vi "Get Access Type.vi"(8 "error in":errorcluster, 11 "Object Entry in":refnum<class "Object Entry.lvclass">) -> (0 "error out":errorcluster, 2 "Access Type":T1=enum."rwr", 3 "Object Entry out":refnum<class "Object Entry.lvclass">)   [LabVIEW 2020, in "CANopen.lvlib" / "Object Entry.lvclass"]
uses:
  Object Entry.lvclass
  Object Entry.lvclass/Object Entry.ctl
  Sub Objects Dictionary/Sub Objects Dictionary.lvclass
  Sub Object/Sub Object.lvclass
  Typedefs/Access Type.ctl
  CANopen.lvlib
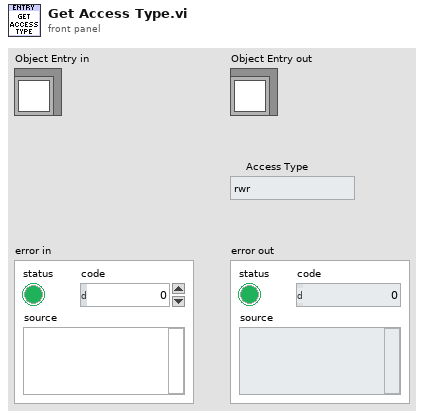
[diagram p1: front panel]
types:
  T1 = typedef "CANopen.lvlib/Access Type.ctl" = enum16{"unknown", "ro", "wo", "rw", "rwr", "rww", "const"}
  T2 = typedef "CANopen.lvlib/Object Type.ctl" = u8
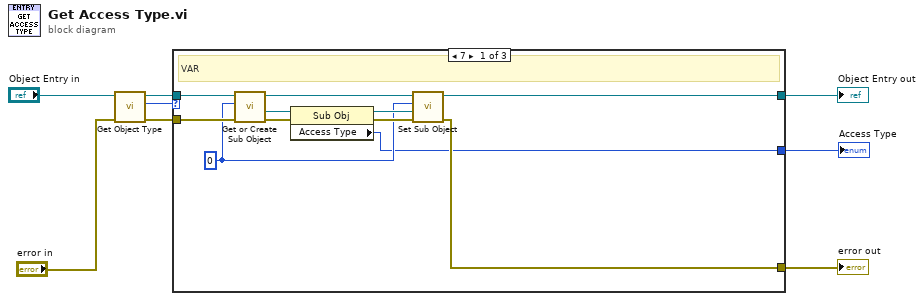
[diagram p0: block diagram]
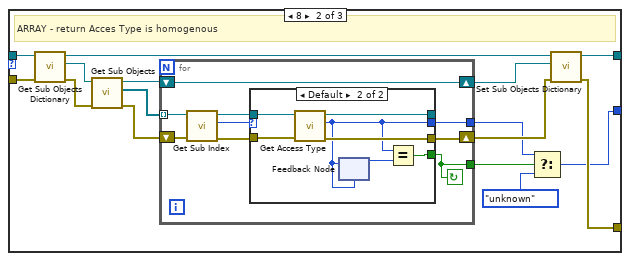
[diagram p2: hidden frame]
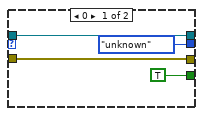
[diagram p3: hidden frame]
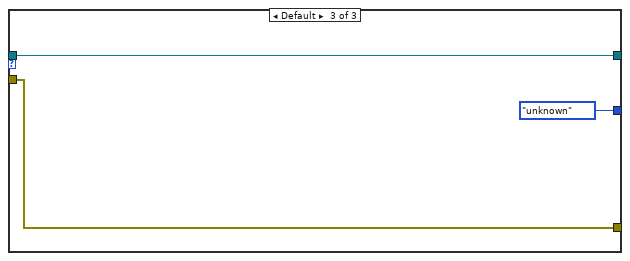
[diagram p4: hidden frame]
diagram:
  n1 = call "Get Object Type.vi"("error in"="error in", "Object Entry in"="Object Entry in") -> ("error out"=w6:errorcluster, "Object Type"=w8:T2, "Object Entry out"=w7:refnum<class "Object Entry.lvclass">)  [unwired: 7 in]
  n2 = case shown="7" w8 {
    tunnel: w7 -> [w19 w33 w57]
    tunnel: w6 -> [w16 w35 w58]
    tunnel: [w12 w24 w58] -> w1
    tunnel: [w11 w27 w57] -> w3
    tunnel: [w9 w20 Access_Type."unknown" ("f")] -> w2
    frame 7 {
      w10 = u8 0 ("Sub Index")
      # "VAR"
      n3 = call "Get or Create Sub Object.vi"("error in"=w16, "Sub Index"=w10, "Obj Entry in"=w19) -> ("error out"=w18:errorcluster, "Sub Object"=w17:refnum<class "Sub Object.lvclass">, "Obj Entry out"=w15:refnum<class "Object Entry.lvclass">)  [unwired: 6 in]
      n4 = property class="Sub Obj"(reference=w17, error in=w18) -> (reference out=w14:refnum<class "Sub Object.lvclass">, error out=w13:errorcluster, "Access Type"=w9:T1)
      n5 = call "Set Sub Object.vi"("error in"=w13, "Sub Object"=w14, "Sub Index"=w10, "Obj Entry in"=w15) -> ("error out"=w12:errorcluster, "Obj Entry out"=w11:refnum<class "Object Entry.lvclass">)  [unwired: 6 in]
    }
    frame 8 {
      # "ARRAY - return Acces Type is homogenous"
      n6 = call "Get Sub Objects Dictionary.vi"("error in"=w35, "Object Entry in"=w33) -> ("error out"=w34:errorcluster, "Sub Objects"=w32:refnum<class "Sub Objects Dictionary.lvclass">, "Object Entry out"=w26:refnum<class "Object Entry.lvclass">)  [unwired: 7 in]
      n7 = call "Get Sub Objects.vi"("error in"=w34, "Sub Objects Dictionary in"=w32) -> ("error out"=w31:errorcluster, "Sub Objects"=w30:refnum<class "Sub Object.lvclass">[], "Sub Objects Dictionary out"=w29:refnum<class "Sub Objects Dictionary.lvclass">)  [unwired: 7 in]
      n8 = for {
        tunnel: w30 -> [w40] mode=indexing
        shift-right: [w43] -> w28
        shift-left: w29 -> [w43]
        shift-right: [w42] -> w25
        shift-left: w31 -> [w44]
        tunnel: [w37] -> w22
        tunnel: [w36] -> w23
        stop <- w36 continue-if-true
        n9 = call "Get Sub Index.vi"("error in"=w44, "Sub Object in"=w40) -> ("error out"=w41:errorcluster, "Sub Index"=w38:u8, "Sub Object out"=w39:refnum<class "Sub Object.lvclass">)  [unwired: 7 in]
        n10 = case shown="Default" w38 {
          tunnel: w39 -> [w48 w55]
          tunnel: w41 -> [w47 w54]
          tunnel: [w48 w53] -> _
          tunnel: [w47 w52] -> w42
          tunnel: [TRUE w50] -> w36
          tunnel: [Access_Type."unknown" ("Access Type") w49] -> w37
          frame 0 {
          }
          frame Default {
            n11 = call "Get Access Type.vi"("error in (no error)"=w54, "Sub Object in"=w55) -> ("error out"=w52:errorcluster, "Access Type"=w49:T1, "Sub Object out"=w53:refnum<class "Sub Object.lvclass">)  [unwired: 7 in]
            n12 = feedback-in #1(w49) -> ()
            n13 = feedback #1(w49) -> (w51:T1)
            n14 = Equal?(x=w49, y=w51) -> (x = y?=w50:bool)
          }
        }
      }
      n15 = Select(t=w22, s=w23, f=Access_Type."unknown") -> (s? t:f=w20:T1)
      n16 = call "Set Sub Objects Dictionary.vi"("error in (no error)"=w25, "Sub Objects Dictionary"=w28, "Object Entry in"=w26) -> ("error out"=w24:errorcluster, "Object Entry out"=w27:refnum<class "Object Entry.lvclass">)  [unwired: 7 in]
    }
    frame Default {
    }
  }
  "error out" <- w1
  "Object Entry out" <- w3
  "Access Type" <- w2
